vi "P9_d7seg.vi"() -> ()   [LabVIEW 2022 SP3]
panel:
  in  "stop":bool
  in  "1\n1":bool
  in  "0":bool
  in  "2":bool
  in  "3":bool
  out "h":bool
  out "f":bool
  out "e":bool
  out "c":bool
  out "b":bool
  out "d":bool
  out "g":bool
  out "a":bool
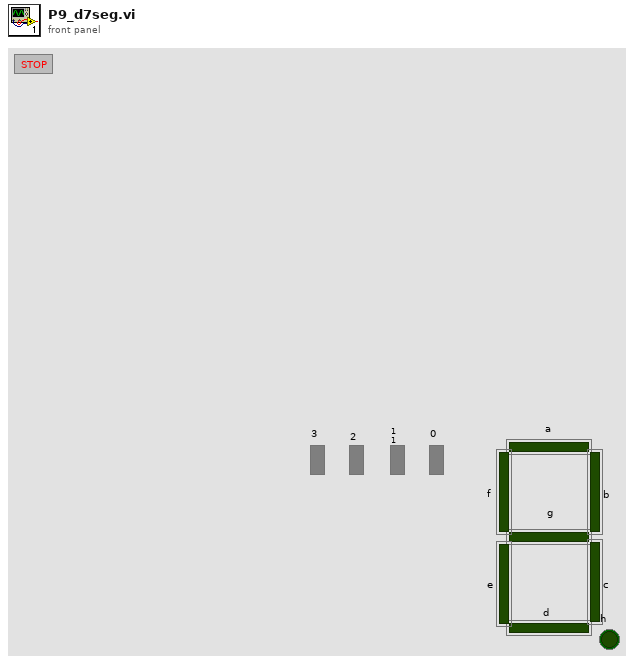
[diagram p1: front panel]
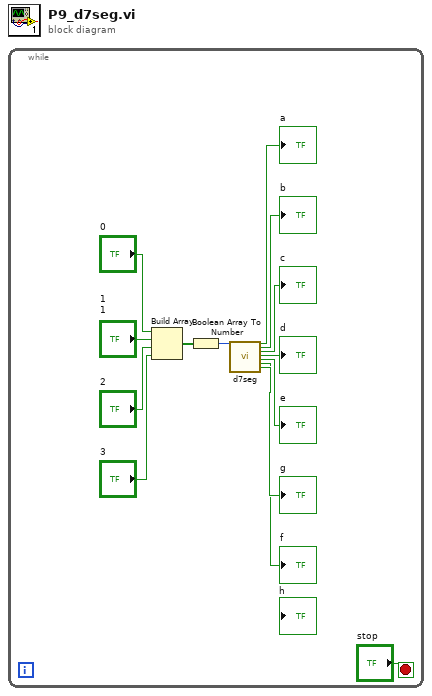
[diagram p0: block diagram]
diagram:
  n1 = while {
    stop <- "stop" stop-if-true
    n2 = Build Array("0", "1\n1", "2", "3") -> (w5:bool[])
    n3 = Boolean Array To Number(Boolean array=w5) -> (number=w4:u32)
    n4 = call "d7seg.vi"("Numeric"=w4) -> ("a"=→"a":bool, "b"=→"b":bool, "c"=→"c":bool, "d"=→"d":bool, "e"=→"e":bool, "f"=→"f":bool, "g"=→"g":bool)  [unwired: 19 in, 1 out]
  }
